vi "Color Get Color Rendering Index.vi"(0 "a_data":dbl[](array[numeric]), 1 "CRI":dbl, 5 "a_CIEResolution":u8, 7 "a_Observer":u8, 9 "R_Values":dbl[](array[numeric]), 11 "error in (no error)":errorcluster) -> (3 "CRI out":dbl, 4 "a_data out":dbl[](array[numeric]), 6 "function return":i16, 10 "R_Values out":dbl[](array[numeric]), 15 "error out":errorcluster)   [LabVIEW 2013, in "AvaSpec.lvlib" / "AVSirrad_support.lvlib" / "AVSirrad.lvlib"]
doc: "DLL_API short int __stdcall Color_GetColorRenderingIndex\n(\n DataType *a_data,\n unsigned char a_CIEResolution,\n unsigned char a_Observer,\n double *R_Values,\n double *CRI\n);"
uses:
  AVSirrad.lvlib
  AVSIRRAD/Examples/Labview/build/AVSirrad.dll
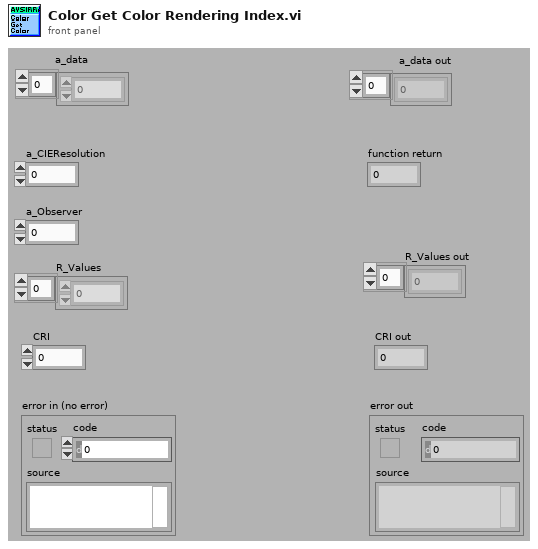
[diagram p1: front panel]
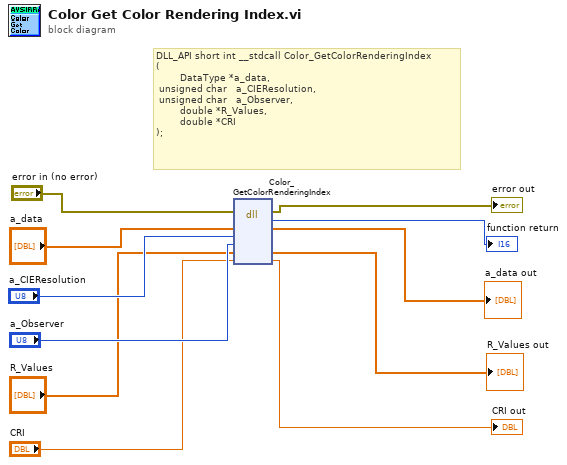
[diagram p0: block diagram]
diagram:
  # "DLL_API short int __stdcall Color_GetColorRenderingIndex\n(\n        DataType *a_data,\n\tunsigned char   a_CIEResolution,\n\tunsigned char   a_Observer,\n        double *R_Values,\n        double *CRI\n);"
  n1 = dll-call lib="C:/AVSIRRAD/Examples/Labview/build/AVSirrad.*" fn="Color_GetColorRenderingIndex"(error in="error in (no error)", "a_data"="a_data", "a_CIEResolution"="a_CIEResolution", "a_Observer"="a_Observer", "R_Values"="R_Values", "CRI"="CRI") -> (error out=→"error out":errorcluster, "return type"=→"function return":i16, "a_data"=→"a_data out":dbl[], "R_Values"=→"R_Values out":dbl[], "CRI"=→"CRI out":dbl)  [unwired: 4 in, 1 out]
